vi "Get Last Error.vi"(8 "error in (no error)":errorcluster, 11 "Nominal Streaming in":refnum<class "Nominal Streaming.lvclass">) -> (0 "error out":errorcluster, 3 "Nominal Streaming out":refnum<class "Nominal Streaming.lvclass">)   [LabVIEW 2020, in "Nominal Streaming.lvclass"]
uses:
  Nominal Streaming.lvclass
  nominal-streaming.bin/nominal_labview_ffi_32.dll
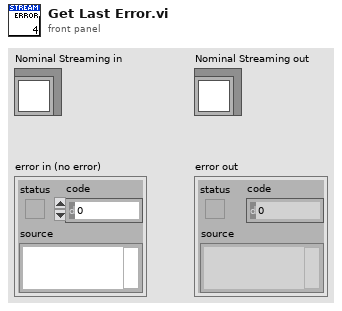
[diagram p1: front panel]
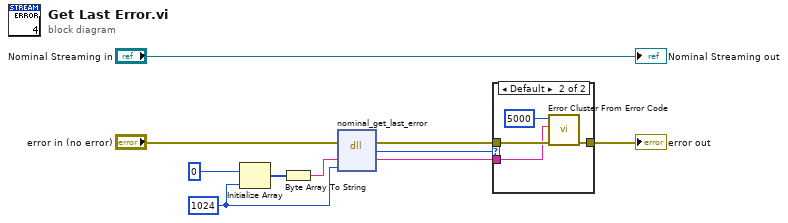
[diagram p0: block diagram]
diagram:
  w9 = u64 1024 ("buffer_size")
  n1 = Initialize Array(u8 0, w9) -> (w8:u8[])
  n2 = Byte Array To String(unsigned byte array=w8) -> (string=w7:string)
  n3 = dll-call lib="C:/code/nominal-streaming-labview-ffi/lv_src/nominal-streaming.bin/nominal_labview_ffi_32.dll" fn="nominal_get_last_error"(error in="error in (no error)", "buffer"=w7, "buffer_size"=w9) -> (error out=w5:errorcluster, "return type"=w1:i32, "buffer"=w3:string)  [unwired: 3 in, 1 out]
  n4 = case shown="Default" w1 {
    tunnel: w5 -> [w11 w15]
    tunnel: [w11 w14] -> w4
    tunnel: w3 -> [_ w13]
    frame -1 {
    }
    frame Default {
      n5 = call <vilib>:"Error Cluster From Error Code.vi"("error in (no error)"=w15, "error message (\"\")"=w13, "error code (0)"=5000) -> ("error out"=w14:errorcluster)  [unwired: 6 in]
    }
  }
  "error out" <- w4
  "Nominal Streaming out" <- "Nominal Streaming in"
